vi "fpga_LineInputsOV-TBank0-0.vi"(5 "overflow":bool) -> (0 "DataLines":T1)   [LabVIEW 2011]
uses:
  <vilib>/rvi/eio/common/nirviEmuTemplateMethod_errors.vi
  <vilib>/eio/EIONode/EIONode.xnode
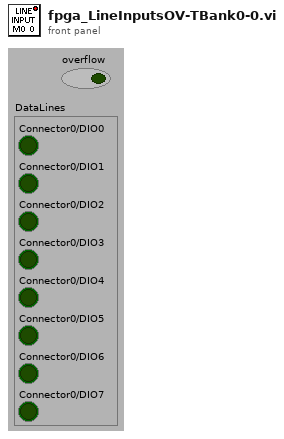
[diagram p1: front panel]
types:
  T1 = cluster{"Connector0/DIO0":bool, "Connector0/DIO1":bool, "Connector0/DIO2":bool, "Connector0/DIO3":bool, "Connector0/DIO4":bool, "Connector0/DIO5":bool, "Connector0/DIO6":bool, "Connector0/DIO7":bool}
  T2 = cluster{bool, bool, bool, bool, bool, bool, bool, bool}
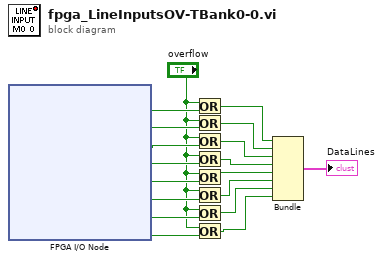
[diagram p0: block diagram]
diagram:
  n1 = xnode "FPGA I/O Node"() -> ("Connector3/DIO22"=w18:bool, "Connector0/DIO4"=w16:bool, "Connector3/DIO21"=w15:bool, "Connector0/DIO8"=w14:bool, "Connector3/DIO23"=w13:bool, "Connector0/DIO6"=w12:bool, "Connector3/DIO16"=w11:bool, "Connector0/DIO5"=w17:bool)  [unwired: 8 in, 8 out]
  n2 = Or(x="overflow", y=w18) -> (x .or. y?=w9:bool)
  n3 = Or(x="overflow", y=w16) -> (x .or. y?=w8:bool)
  n4 = Or(x="overflow", y=w15) -> (x .or. y?=w7:bool)
  n5 = Or(x="overflow", y=w14) -> (x .or. y?=w6:bool)
  n6 = Or(x="overflow", y=w13) -> (x .or. y?=w5:bool)
  n7 = Or(x="overflow", y=w12) -> (x .or. y?=w4:bool)
  n8 = Or(x="overflow", y=w11) -> (x .or. y?=w3:bool)
  n9 = Or(x="overflow", y=w17) -> (x .or. y?=w2:bool)
  n10 = Bundle(w9, w8, w7, w6, w5, w4, w3, w2) -> (→"DataLines":T2)  [unwired: 1 in]
